vi "memory_load_MLP_2_C_1.vi"() -> ()   [LabVIEW 2020]
panel:
  out "appended path":path
  out "Array":fxp<+/-,32,16>[](array[numeric])
  out "Init Data Out":fxp<+/-,32,16>[][](array[numeric])
  out "size(s)":i32
  # "For Initialization VI requirements and help, please read directions located on Block Diagram."
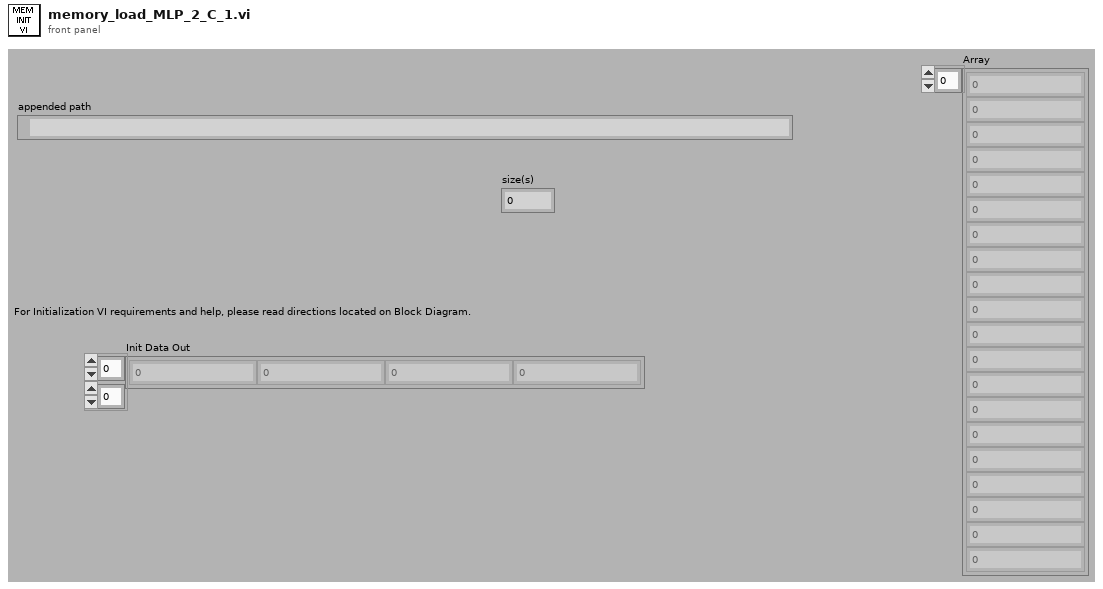
[diagram p1: front panel]
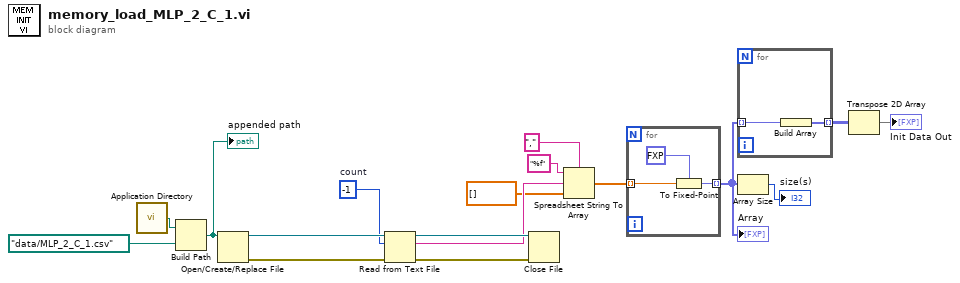
[diagram p0: block diagram]
diagram:
  w4 = -1  # count
  n1 = call <vilib>:"Application Directory.vi"() -> ("Application Directory"=w8:path)
  n2 = Build Path(base path=w8, name or relative path=path "data/MLP_2_C_1.csv" ("default name")) -> (appended path=w7:path)
  "appended path" <- w7
  n3 = Open/Create/Replace File(file path (use dialog)=w7) -> (refnum out=w12:refnum<file>, error out=w13:errorcluster)  [unwired: 5 in, 1 out]
  n4 = Read from Text File(file (use dialog)=w12, count=w4, error in=w13) -> (refnum out=w11:refnum<file>, text=w9:string, error out=w10:errorcluster)  [unwired: 1 in, 1 out]
  n5 = Close File(refnum=w11, error in=w10) -> ()  [unwired: 2 out]
  n6 = Spreadsheet String To Array(delimiter (Tab)=",", format string="%f", spreadsheet string=w9, array type (2D Dbl)=dbl[] []) -> (array=w1:dbl[])
  n7 = for {
    tunnel: w1 -> [w20] mode=indexing
    tunnel: [w19] -> w16 mode=indexing
    n8 = To Fixed-Point(fixed-point type=fxp<+/-,32,16> 0.0 ("fixed-point"), number=w20) -> (fixed-point=w19:fxp<+/-,32,16>)
  }
  "Array" <- w16
  n9 = for {
    tunnel: w16 -> [w22] mode=indexing
    tunnel: [w21] -> w15 mode=indexing
    n10 = Build Array(w22) -> (w21:fxp<+/-,32,16>[])
  }
  n11 = Array Size(array=w16) -> (size(s)=→"size(s)":i32)
  n12 = Transpose 2D Array(2D array=w15) -> (transposed array=→"Init Data Out":fxp<+/-,32,16>[][])
